vi "Miniquads.ProcCases.vi"(0 "i ref in":refnum<vi>, 1 "selector":string, 2 "Data":T1, 3 "call cluster":T2={"Object"="", "Selector"="", "CallType"=enum."synchronous", "Async Object"="", "Async Selector"="", "Data Descriptor"="", "Data"=[], "Error #"=0, "Expire"=0}, 5 "error in (no error)":errorcluster) -> (14 "i ref out":refnum<vi>, 17 "answer cluster":T2={"Object"="", "Selector"="", "CallType"=enum."synchronous", "Async Object"="", "Async Selector"="", "Data Descriptor"="", "Data"=[], "Error #"=0, "Expire"=0}, 19 "error out":errorcluster)   [LabVIEW 2014, in "Miniquads.lvlib"]
doc: "This method is called by a process from within the default case in the event loop. The methods of a class that are linked to events will be called from THIS method. Add your code here."
uses:
  Miniquads.lvlib
  CS_Core/CSSystem/CoreDefs/CoreDefs.call_type.ctl
  CS_Core/BaseProcess/BaseProcess.descriptor string definition.ctl
  CS_Core/CSSystem/CoreDefs/CoreDefs.rawDataType.ctl
  CS_Core/CSSystem/CoreLib/CoreLib.byte array 2 double.vi
  CS_Core/CSSystem/CoreLib/CoreLib.double 2 byte array.vi
  CS_Core/CSSystem/CoreLib/CoreLib.string 2 byte array.vi
  CS_Core/CSSystem/CoreLib/CoreLib.lvlib
  CS_Core/BaseProcess/BaseProcess.lvlib
  CS_Core/CSApplicationBaseClasses/DeviceBase/DeviceBase.lvlib
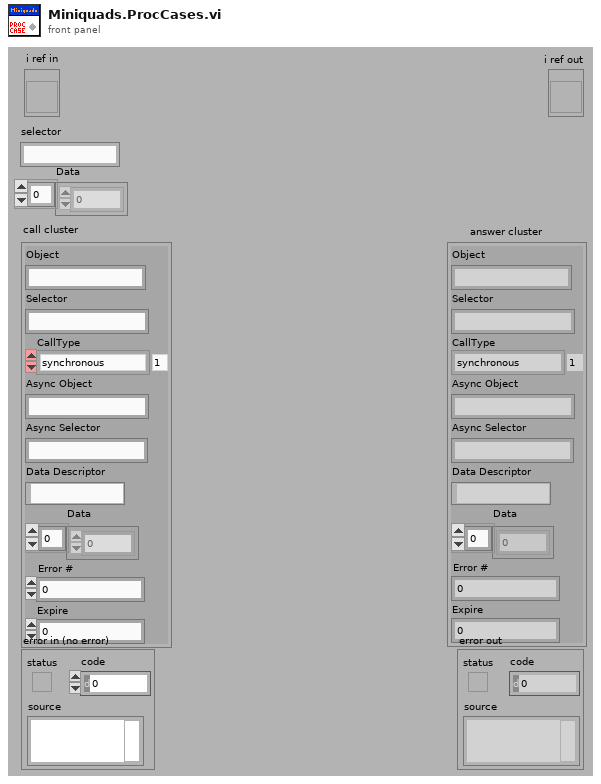
[diagram p1: front panel]
types:
  T1 = typedef "CoreDefs.rawDataType.ctl" = i8[]
  T2 = typedef "CoreDefs.call_type.ctl" = cluster{"Object":string, "Selector":string, "CallType":enum16{"simple", "synchronous", "asynchronous"}, "Async Object":string, "Async Selector":string, "Data Descriptor":T3, "Data":T1, "Error #":i32, "Expire":u32}
  T3 = typedef "BaseProcess.lvlib/BaseProcess.descriptor string definition.ctl" = string
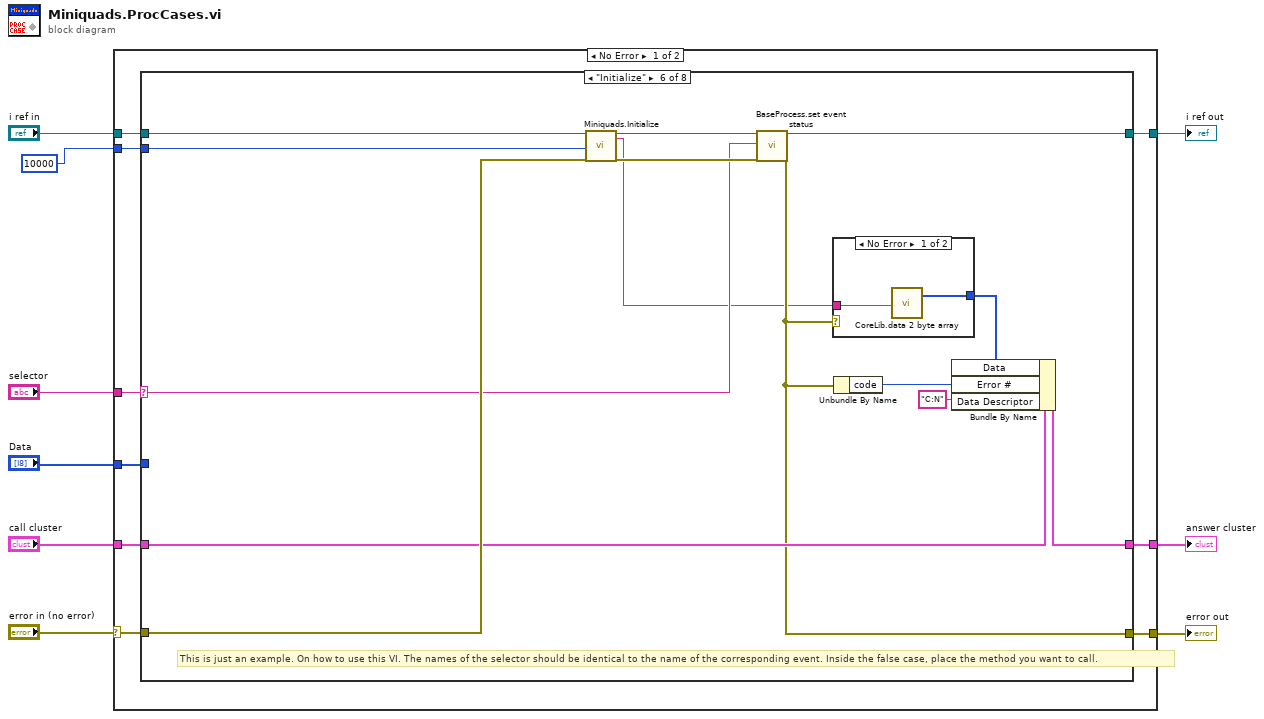
[diagram p0: block diagram]
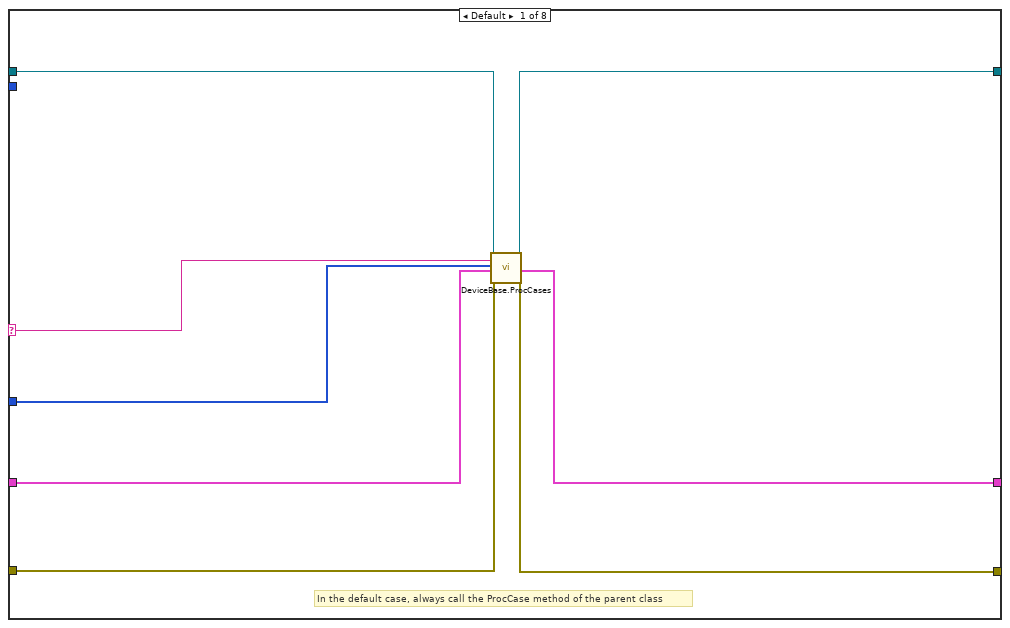
[diagram p2: hidden frame]
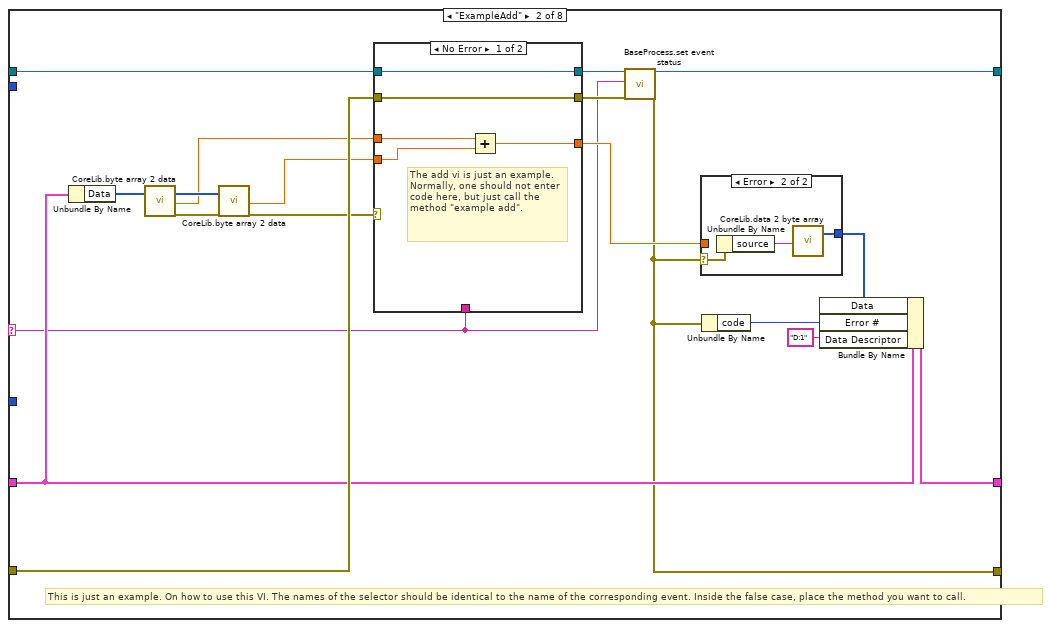
[diagram p3: hidden frame]
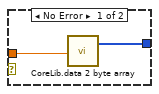
[diagram p4: hidden frame]
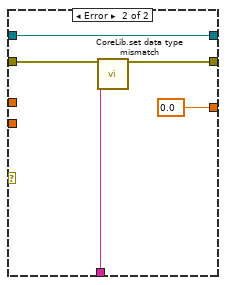
[diagram p5: hidden frame]
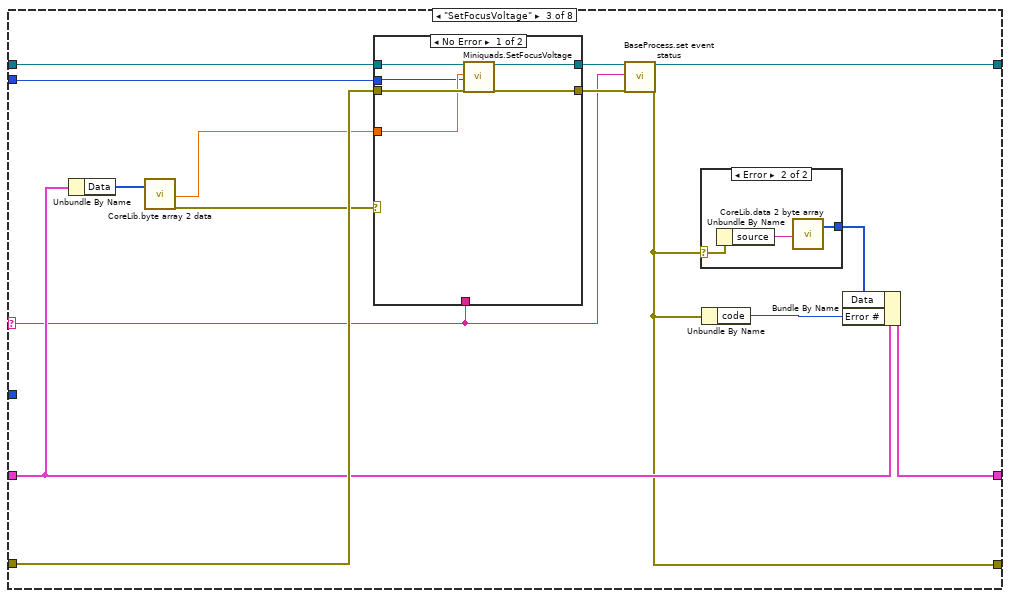
[diagram p6: hidden frame]
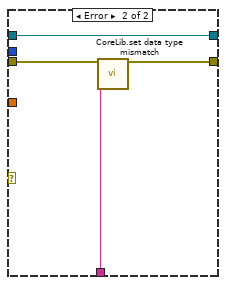
[diagram p8: hidden frame]
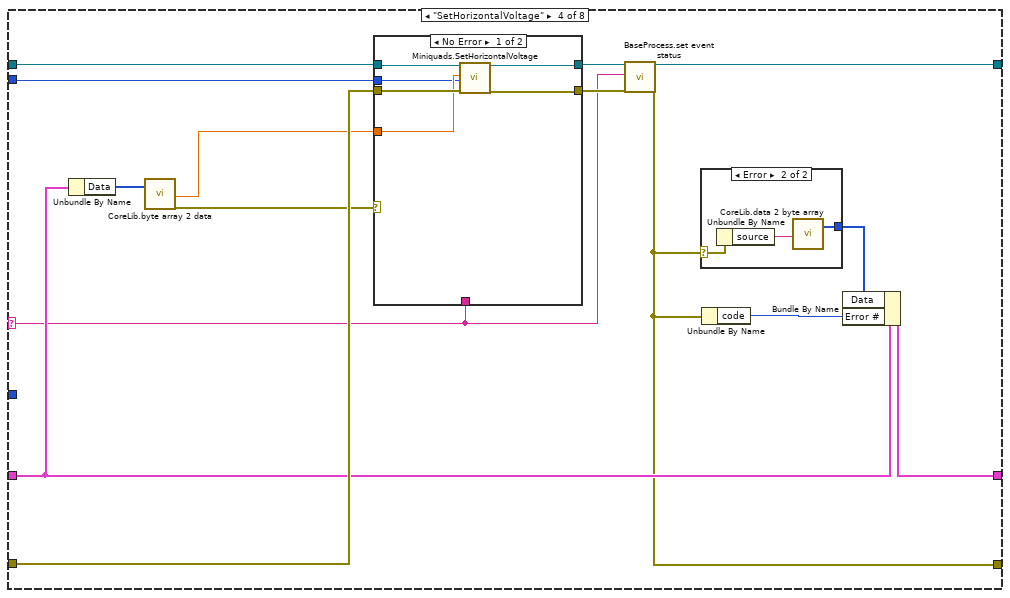
[diagram p9: hidden frame]
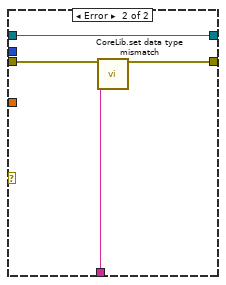
[diagram p11: hidden frame]
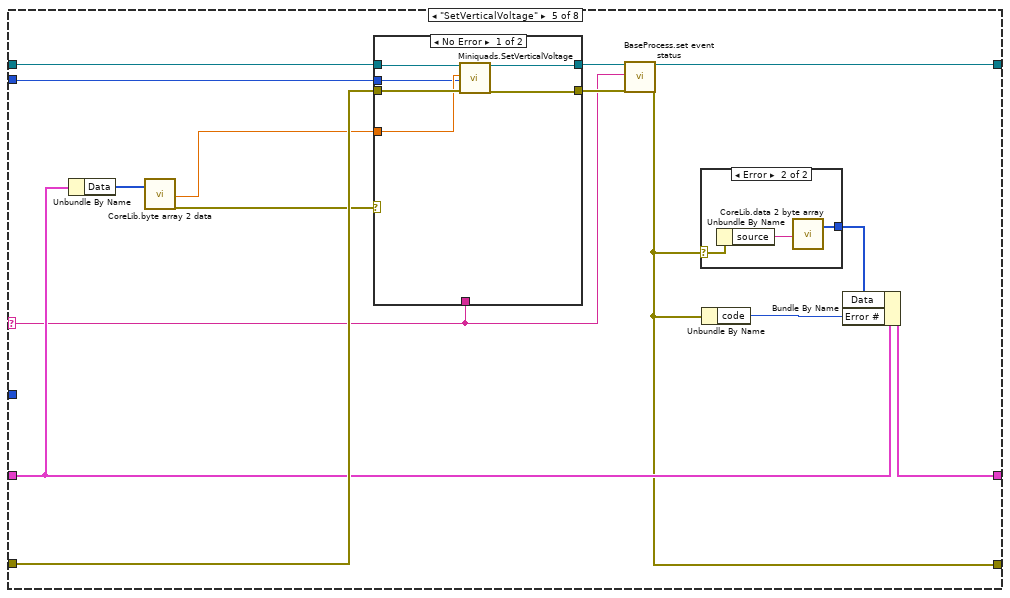
[diagram p12: hidden frame]
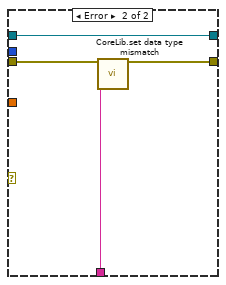
[diagram p14: hidden frame]
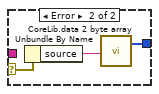
[diagram p15: hidden frame]
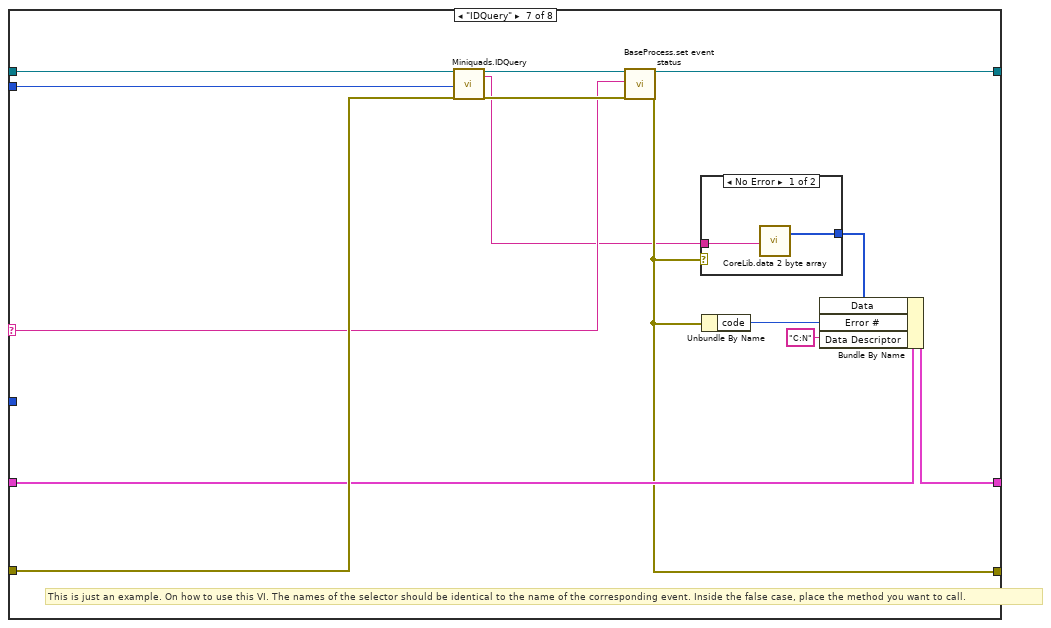
[diagram p16: hidden frame]
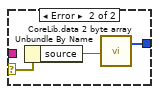
[diagram p17: hidden frame]
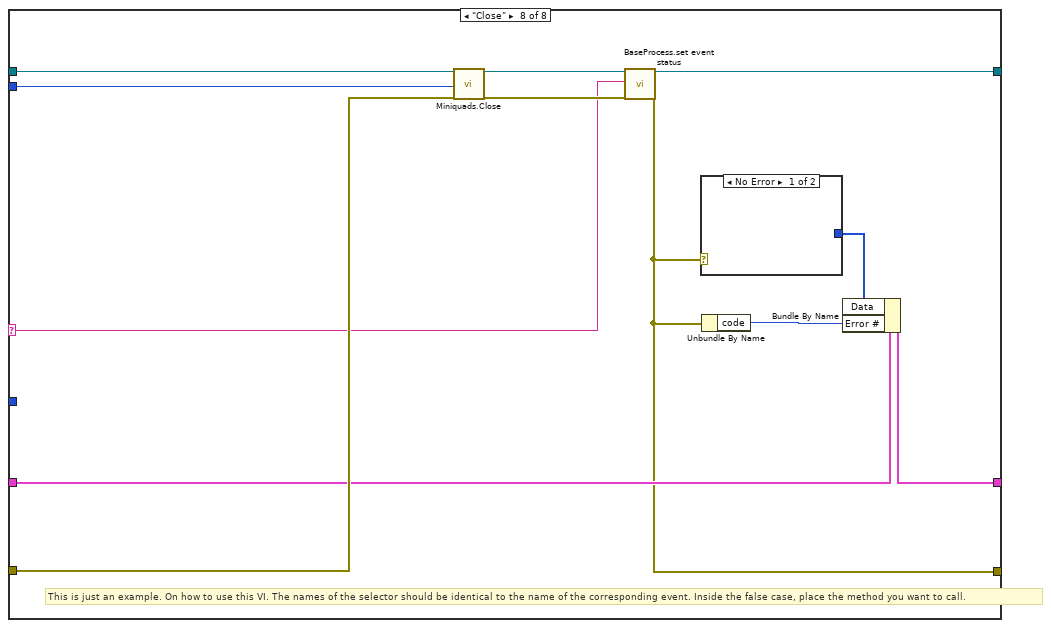
[diagram p18: hidden frame]
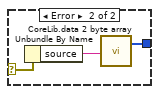
[diagram p19: hidden frame]
diagram:
  n1 = case shown="No Error" "error in (no error)" {
    selector: "error in (no error)" -> [w11 w198]
    tunnel: "selector" -> [w18 _]
    tunnel: [w17 w199] -> w8
    tunnel: "Data" -> [w16 _]
    tunnel: "call cluster" -> [w15 w199]
    tunnel: "i ref in" -> [w14 w200]
    tunnel: [w13 w200] -> w4
    tunnel: [w12 w198] -> w3
    tunnel: 10000 ("ms timeout (10000)") -> [w10 _]
    frame No Error {
      n2 = case shown="\"Initialize\"" w18 {
        selector: w18 -> [w21 w35 w66 w94 w122 w149 w168 w185]
        tunnel: w16 -> [w19 _ _ _ _ _ _ _]
        tunnel: w14 -> [w20 w45 w75 w103 w131 w158 w177 w194]
        tunnel: [w26 w34 w65 w93 w121 w148 w167 w184] -> w13
        tunnel: w15 -> [w22 w41 w72 w100 w128 w155 w174 w191]
        tunnel: [w23 w40 w71 w99 w127 w154 w173 w190] -> w17
        tunnel: w11 -> [w25 w44 w74 w102 w130 w157 w176 w193]
        tunnel: [w24 w36 w67 w95 w123 w150 w169 w186] -> w12
        tunnel: w10 -> [_ _ w61 w89 w117 w145 w164 w183]
        frame Default {
          # "In the default case, always call the ProcCase method of the parent class"
          n3 = call "DeviceBase.ProcCases.vi"("i ref in"=w20, "selector"=w21, "Data"=w19, "call cluster"=w22, "error in (no error)"=w25) -> ("i ref out"=w26:refnum<vi>, "answer cluster"=w23:T2, "error out"=w24:errorcluster)  [unwired: 12 in]
        }
        frame "ExampleAdd" {
          # "This is just an example. On how to use this VI. The names of the selector should be identical to the name of the corresponding event. Inside the false case, place the method you want to call."
          n4 = Unbundle By Name(w41) -> ("Data"=w32:T1)
          n5 = call-poly "CoreLib.byte array 2 data.vi"("byteArray"=w32) -> ("byteArray out"=w30:T1, "d64"=w28:dbl, "error out"=w31:errorcluster)  [unwired: 16 in]
          n6 = call-poly "CoreLib.byte array 2 data.vi"("byteArray"=w30, "error in (no error)"=w31) -> ("d64"=w27:dbl, "error out"=w29:errorcluster)  [unwired: 15 in, 1 out]
          n7 = case shown="No Error" w29 {
            tunnel: [w52 w60] -> w38
            tunnel: w45 -> [w52 w60]
            tunnel: w44 -> [w53 w59]
            tunnel: [w53 w58] -> w37
            tunnel: w27 -> [w55 _]
            tunnel: [w54 0.0] -> w43
            tunnel: w35 -> [_ w56]
            tunnel: w28 -> [w51 _]
            frame No Error {
              # "The add vi is just an example. Normally, one should not enter code here, but just call the method \"example add\"."
              n8 = Add(x=w51, y=w55) -> (x+y=w54:dbl)
            }
            frame Error {
              n9 = call "CoreLib.set data type mismatch.vi"("error in (no error)"=w59, "error source"=w56) -> ("error out"=w58:errorcluster)  [unwired: 17 in]
            }
          }
          n10 = call "BaseProcess.set event status.vi"("i ref in"=w38, "EventStatus"=w35, "error in (no error)"=w37) -> ("i ref out"=w34:refnum<vi>, "error out"=w36:errorcluster)  [unwired: 14 in, 1 out]
          n11 = case shown="Error" w36 {
            selector: w36 -> [_ w50]
            tunnel: [w46 w49] -> w39
            tunnel: w43 -> [w47 _]
            frame No Error {
              n12 = call-poly "CoreLib.data 2 byte array.vi"("f64"=w47) -> ("byteArray out"=w46:T1)  [unwired: 18 in]
            }
            frame Error {
              n13 = Unbundle By Name(w50) -> ("source"=w48:string)
              n14 = call-poly "CoreLib.data 2 byte array.vi"("string"=w48) -> ("byteArray out"=w49:T1)  [unwired: 18 in]
            }
          }
          n15 = Unbundle By Name(w36) -> ("code"=w42:i32)
          n16 = Bundle By Name(cluster=w41, "Data"=w39, "Error #"=w42, "Data Descriptor"="D:1") -> (w40:T2)
        }
        frame "SetFocusVoltage" {
          n17 = Unbundle By Name(w72) -> ("Data"=w64:T1)
          n18 = call-poly "CoreLib.byte array 2 data.vi"("byteArray"=w64) -> ("d64"=w63:dbl, "error out"=w62:errorcluster)  [unwired: 16 in, 1 out]
          n19 = case shown="No Error" w62 {
            tunnel: [w83 w88] -> w69
            tunnel: w75 -> [w84 w88]
            tunnel: w74 -> [w81 w87]
            tunnel: [w82 w86] -> w68
            tunnel: w66 -> [_ w85]
            tunnel: w63 -> [w80 _]
            tunnel: w61 -> [w79 _]
            frame No Error {
              n20 = call "Miniquads.SetFocusVoltage.vi"("i ref in"=w84, "FocusVoltage"=w80, "ms timeout (10000)"=w79, "error in (no error)"=w81) -> ("i ref out"=w83:refnum<vi>, "error out"=w82:errorcluster)  [unwired: 13 in, 1 out]
            }
            frame Error {
              n21 = call "CoreLib.set data type mismatch.vi"("error in (no error)"=w87, "error source"=w85) -> ("error out"=w86:errorcluster)  [unwired: 17 in]
            }
          }
          n22 = call "BaseProcess.set event status.vi"("i ref in"=w69, "EventStatus"=w66, "error in (no error)"=w68) -> ("i ref out"=w65:refnum<vi>, "error out"=w67:errorcluster)  [unwired: 14 in, 1 out]
          n23 = case shown="Error" w67 {
            selector: w67 -> [_ w78]
            tunnel: [_ w77] -> w70
            frame No Error {
            }
            frame Error {
              n24 = Unbundle By Name(w78) -> ("source"=w76:string)
              n25 = call-poly "CoreLib.data 2 byte array.vi"("string"=w76) -> ("byteArray out"=w77:T1)  [unwired: 18 in]
            }
          }
          n26 = Unbundle By Name(w67) -> ("code"=w73:i32)
          n27 = Bundle By Name(cluster=w72, "Data"=w70, "Error #"=w73) -> (w71:T2)
        }
        frame "SetHorizontalVoltage" {
          n28 = Unbundle By Name(w100) -> ("Data"=w92:T1)
          n29 = call-poly "CoreLib.byte array 2 data.vi"("byteArray"=w92) -> ("d64"=w91:dbl, "error out"=w90:errorcluster)  [unwired: 16 in, 1 out]
          n30 = case shown="No Error" w90 {
            tunnel: [w109 w116] -> w97
            tunnel: w103 -> [w110 w116]
            tunnel: w102 -> [w111 w115]
            tunnel: [w112 w114] -> w96
            tunnel: w94 -> [_ w113]
            tunnel: w91 -> [w108 _]
            tunnel: w89 -> [w107 _]
            frame No Error {
              n31 = call "Miniquads.SetHorizontalVoltage.vi"("i ref in"=w110, "HorizontalVoltage"=w108, "ms timeout (10000)"=w107, "error in (no error)"=w111) -> ("i ref out"=w109:refnum<vi>, "error out"=w112:errorcluster)  [unwired: 13 in, 1 out]
            }
            frame Error {
              n32 = call "CoreLib.set data type mismatch.vi"("error in (no error)"=w115, "error source"=w113) -> ("error out"=w114:errorcluster)  [unwired: 17 in]
            }
          }
          n33 = call "BaseProcess.set event status.vi"("i ref in"=w97, "EventStatus"=w94, "error in (no error)"=w96) -> ("i ref out"=w93:refnum<vi>, "error out"=w95:errorcluster)  [unwired: 14 in, 1 out]
          n34 = case shown="Error" w95 {
            selector: w95 -> [_ w106]
            tunnel: [_ w105] -> w98
            frame No Error {
            }
            frame Error {
              n35 = Unbundle By Name(w106) -> ("source"=w104:string)
              n36 = call-poly "CoreLib.data 2 byte array.vi"("string"=w104) -> ("byteArray out"=w105:T1)  [unwired: 18 in]
            }
          }
          n37 = Unbundle By Name(w95) -> ("code"=w101:i32)
          n38 = Bundle By Name(cluster=w100, "Data"=w98, "Error #"=w101) -> (w99:T2)
        }
        frame "SetVerticalVoltage" {
          n39 = Unbundle By Name(w128) -> ("Data"=w120:T1)
          n40 = call-poly "CoreLib.byte array 2 data.vi"("byteArray"=w120) -> ("d64"=w119:dbl, "error out"=w118:errorcluster)  [unwired: 16 in, 1 out]
          n41 = case shown="No Error" w118 {
            tunnel: [w137 w144] -> w125
            tunnel: w131 -> [w138 w144]
            tunnel: w130 -> [w139 w143]
            tunnel: [w140 w142] -> w124
            tunnel: w122 -> [_ w141]
            tunnel: w119 -> [w136 _]
            tunnel: w117 -> [w135 _]
            frame No Error {
              n42 = call "Miniquads.SetVerticalVoltage.vi"("i ref in"=w138, "VerticalVoltage"=w136, "ms timeout (10000)"=w135, "error in (no error)"=w139) -> ("i ref out"=w137:refnum<vi>, "error out"=w140:errorcluster)  [unwired: 13 in, 1 out]
            }
            frame Error {
              n43 = call "CoreLib.set data type mismatch.vi"("error in (no error)"=w143, "error source"=w141) -> ("error out"=w142:errorcluster)  [unwired: 17 in]
            }
          }
          n44 = call "BaseProcess.set event status.vi"("i ref in"=w125, "EventStatus"=w122, "error in (no error)"=w124) -> ("i ref out"=w121:refnum<vi>, "error out"=w123:errorcluster)  [unwired: 14 in, 1 out]
          n45 = case shown="Error" w123 {
            selector: w123 -> [_ w134]
            tunnel: [_ w133] -> w126
            frame No Error {
            }
            frame Error {
              n46 = Unbundle By Name(w134) -> ("source"=w132:string)
              n47 = call-poly "CoreLib.data 2 byte array.vi"("string"=w132) -> ("byteArray out"=w133:T1)  [unwired: 18 in]
            }
          }
          n48 = Unbundle By Name(w123) -> ("code"=w129:i32)
          n49 = Bundle By Name(cluster=w128, "Data"=w126, "Error #"=w129) -> (w127:T2)
        }
        frame "Initialize" {
          # "This is just an example. On how to use this VI. The names of the selector should be identical to the name of the corresponding event. Inside the false case, place the method you want to call."
          n50 = call "Miniquads.Initialize.vi"("i ref in"=w158, "ms timeout (10000)"=w145, "error in (no error)"=w157) -> ("i ref out"=w152:refnum<vi>, "DeviceID"=w146:string, "error out"=w151:errorcluster)  [unwired: 13 in, 1 out]
          n51 = call "BaseProcess.set event status.vi"("i ref in"=w152, "EventStatus"=w149, "error in (no error)"=w151) -> ("i ref out"=w148:refnum<vi>, "error out"=w150:errorcluster)  [unwired: 14 in, 1 out]
          n52 = case shown="No Error" w150 {
            selector: w150 -> [_ w163]
            tunnel: [w159 w162] -> w153
            tunnel: w146 -> [w160 _]
            frame No Error {
              n53 = call-poly "CoreLib.data 2 byte array.vi"("string"=w160) -> ("byteArray out"=w159:T1)  [unwired: 18 in]
            }
            frame Error {
              n54 = Unbundle By Name(w163) -> ("source"=w161:string)
              n55 = call-poly "CoreLib.data 2 byte array.vi"("string"=w161) -> ("byteArray out"=w162:T1)  [unwired: 18 in]
            }
          }
          n56 = Unbundle By Name(w150) -> ("code"=w156:i32)
          n57 = Bundle By Name(cluster=w155, "Data"=w153, "Error #"=w156, "Data Descriptor"="C:N") -> (w154:T2)
        }
        frame "IDQuery" {
          # "This is just an example. On how to use this VI. The names of the selector should be identical to the name of the corresponding event. Inside the false case, place the method you want to call."
          n58 = call "Miniquads.IDQuery.vi"("i ref in"=w177, "ms timeout (10000)"=w164, "error in (no error)"=w176) -> ("i ref out"=w171:refnum<vi>, "DeviceID"=w165:string, "error out"=w170:errorcluster)  [unwired: 13 in, 1 out]
          n59 = call "BaseProcess.set event status.vi"("i ref in"=w171, "EventStatus"=w168, "error in (no error)"=w170) -> ("i ref out"=w167:refnum<vi>, "error out"=w169:errorcluster)  [unwired: 14 in, 1 out]
          n60 = case shown="No Error" w169 {
            selector: w169 -> [_ w182]
            tunnel: [w178 w181] -> w172
            tunnel: w165 -> [w179 _]
            frame No Error {
              n61 = call-poly "CoreLib.data 2 byte array.vi"("string"=w179) -> ("byteArray out"=w178:T1)  [unwired: 18 in]
            }
            frame Error {
              n62 = Unbundle By Name(w182) -> ("source"=w180:string)
              n63 = call-poly "CoreLib.data 2 byte array.vi"("string"=w180) -> ("byteArray out"=w181:T1)  [unwired: 18 in]
            }
          }
          n64 = Unbundle By Name(w169) -> ("code"=w175:i32)
          n65 = Bundle By Name(cluster=w174, "Data"=w172, "Error #"=w175, "Data Descriptor"="C:N") -> (w173:T2)
        }
        frame "Close" {
          # "This is just an example. On how to use this VI. The names of the selector should be identical to the name of the corresponding event. Inside the false case, place the method you want to call."
          n66 = call "Miniquads.Close.vi"("i ref in"=w194, "ms timeout (10000)"=w183, "error in (no error)"=w193) -> ("i ref out"=w188:refnum<vi>, "error out"=w187:errorcluster)  [unwired: 14 in, 1 out]
          n67 = call "BaseProcess.set event status.vi"("i ref in"=w188, "EventStatus"=w185, "error in (no error)"=w187) -> ("i ref out"=w184:refnum<vi>, "error out"=w186:errorcluster)  [unwired: 14 in, 1 out]
          n68 = case shown="No Error" w186 {
            selector: w186 -> [_ w197]
            tunnel: [_ w196] -> w189
            frame No Error {
            }
            frame Error {
              n69 = Unbundle By Name(w197) -> ("source"=w195:string)
              n70 = call-poly "CoreLib.data 2 byte array.vi"("string"=w195) -> ("byteArray out"=w196:T1)  [unwired: 18 in]
            }
          }
          n71 = Unbundle By Name(w186) -> ("code"=w192:i32)
          n72 = Bundle By Name(cluster=w191, "Data"=w189, "Error #"=w192) -> (w190:T2)
        }
      }
    }
    frame Error {
    }
  }
  "answer cluster" <- w8
  "i ref out" <- w4
  "error out" <- w3
